vi "ST5 Settings Mess.vi"(8 "error in (no error)":errorcluster, 9 "Actuator names":string[](array[string]), 11 "Name":string) -> (0 "error out":errorcluster, 1 "Cancel Out":bool, 3 "Name Out":string)   [LabVIEW 2019]
doc: "Use this template to build a VI to use as a subVI."
panel:
  in  "Cancel Button":bool
  in  "OK Button":bool
  # "Save Setting"
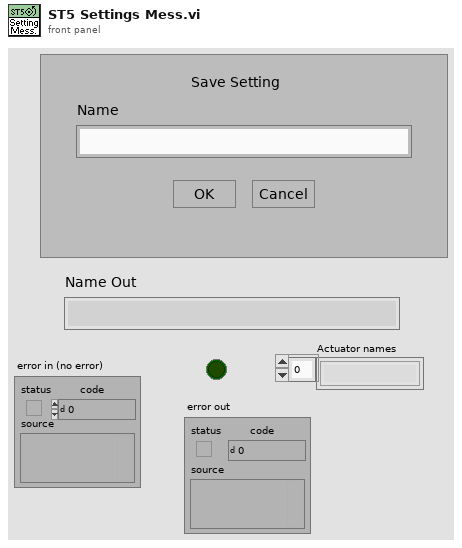
[diagram p1: front panel]
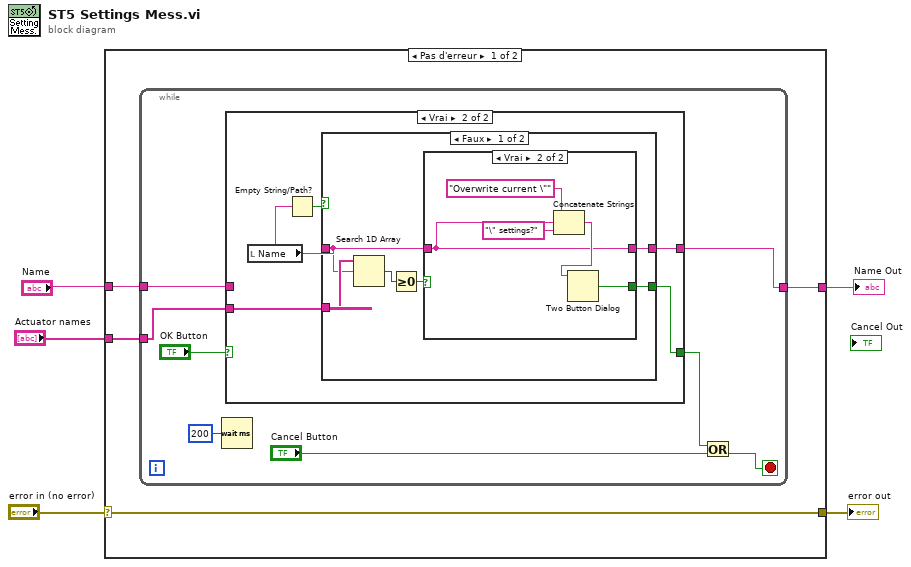
[diagram p0: block diagram]
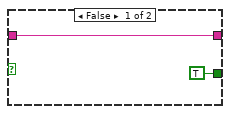
[diagram p3: hidden frame]
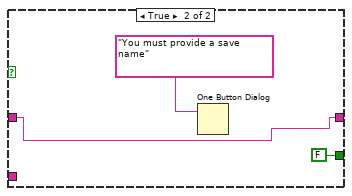
[diagram p4: hidden frame]
diagram:
  n1 = case shown="Pas d'erreur" "error in (no error)" {
    selector: "error in (no error)" -> [w7 w41]
    tunnel: [w7 w41] -> w4
    tunnel: [w9 _] -> w3
    tunnel: "Name" -> [w8 _]
    tunnel: "Actuator names" -> [w6 _]
    frame No Error {
      n2 = while {
        tunnel: [w11] -> w9
        tunnel: w8 -> [w12]
        tunnel: w6 -> [w10]
        stop <- w15 stop-if-true
        n3 = Wait (ms)(milliseconds to wait=u32 200) -> ()  [unwired: 1 out]
        n4 = case shown="Vrai" "OK Button" {
          selector: "OK Button" -> [w19 _]
          tunnel: [w19 w24] -> w13
          tunnel: w12 -> [w18 _]
          tunnel: [w18 w23] -> w11
          tunnel: w10 -> [_ w20]
          frame False {
          }
          frame True {
            n5 = local read "Name"() -> (w21:string)
            n6 = Empty String/Path?(string/path=w21) -> (empty?=w22:bool)
            n7 = case shown="Faux" w22 {
              tunnel: [w30 FALSE ("T button?")] -> w24
              tunnel: [w29 w38] -> w23
              tunnel: w21 -> [w27 w38]
              tunnel: w20 -> [w28 _]
              frame False {
                n8 = Search 1D Array(1D array=w28, element=w27) -> (index of element=w25:i32)  [unwired: 1 in]
                n9 = Greater Or Equal To 0?(x=w25) -> (x >= 0?=w26:bool)
                n10 = case shown="Vrai" w26 {
                  tunnel: w27 -> [w31 w33]
                  tunnel: [TRUE ("T button?") w34] -> w30
                  tunnel: [w31 w33] -> w29
                  frame False {
                  }
                  frame True {
                    n11 = Concatenate Strings("Overwrite current \"", w33, "\" settings?" ("string")) -> (w35:string)
                    n12 = Two Button Dialog(message=w35) -> (T button?=w34:bool)  [unwired: 2 in]
                  }
                }
              }
              frame True {
                n13 = One Button Dialog(message="You must provide a save name") -> ()  [unwired: 1 in, 1 out]
              }
            }
          }
        }
        n14 = Or(x=w13, y="Cancel Button") -> (x .or. y?=w15:bool)
      }
    }
    frame Error {
    }
  }
  "error out" <- w4
  "Name Out" <- w3
